vi "AustinWeatherParse.vi"(11 "file path (dialog if empty)":path) -> (2 "Year":i32[](array[numeric]), 3 "Average Temp Array":dbl[](array[numeric]))   [LabVIEW 2014]
uses:
  <vilib>/Utility/file.llb/Read From Spreadsheet File (string).vi
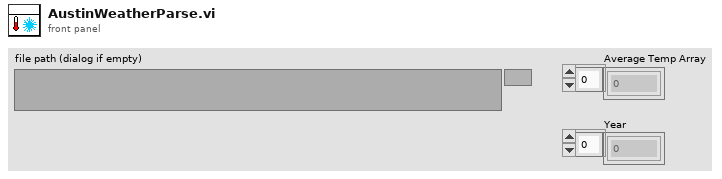
[diagram p1: front panel]
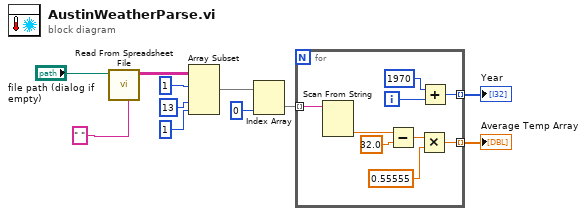
[diagram p0: block diagram]
diagram:
  n1 = call-poly <vilib>:"Read From Spreadsheet File.vi"("delimiter (\\t)"=" " ("delimiter (\\t)"), "file path (dialog if empty)"="file path (dialog if empty)") -> ("all rows"=w3:string[][])  [unwired: 5 in, 4 out]
  n2 = Array Subset(array=w3, index (row)=1 ("index"), index (col)=13 ("index"), length (col)=1 ("length")) -> (w7:string[][])  [unwired: 1 in]
  n3 = Index Array(array=w7, index (col)=0 ("disabled index (col)")) -> (element=w9:string[])  [unwired: 1 in]
  n4 = for {
    tunnel: w9 -> [w20] mode=indexing
    tunnel: [w15] -> w11 mode=indexing
    tunnel: [w12] -> w10 mode=indexing
    i -> [w14]
    n5 = Scan From String(input string=w20) -> (output 1=w18:dbl)  [unwired: 4 in, 3 out]
    n6 = Subtract(x=w18, y=32.0) -> (x-y=w16:dbl)
    n7 = Multiply(x=w16, y=0.55555) -> (x*y=w15:dbl)
    n8 = Add(x=1970, y=w14) -> (x+y=w12:i32)
  }
  "Average Temp Array" <- w11
  "Year" <- w10
